vi "Detect PSw.vi"(4 "Contralateral Event Data":T1={"Event Data"={"LR"={"Phase"="LR", "On"=FALSE, "Last On Time"=0.0, "Duration"=0.0, "Crossing Time"=0.0, "Time since LR"=0.0, "Time Since TSw"=0.0, "Min gyro Z"=0.0, "Time since LR?"=FALSE, "Time since TSw?"=FALSE, "Min gyro Z?"=FALSE, "Crossing?"=FALSE}, "MSt"={"Phase"="MSt", "On"=FALSE, "Last On Time"=0.0, "Duration"=0.0}, "TSt"={"Phase"="TSt", "On"=FALSE, "Last On Time"=0.0, "Duration"=0.0}, "PSw"={"Phase"="PSw", "On"=FALSE, "Last On Time"=0.0, "Duration"=0.0}, "ISw"={"Phase"="ISw", "On"=FALSE, "Last On Time"=0.0, "Duration"=0.0, "Peak Time"=0.0, "Time since LR"=0.0, "Time since ISw"=0.0, "Time since LR?"=FALSE, "Time since ISw?"=FALSE, "Peak?"=FALSE}, "MSw"={"Phase"="MSw", "On"=FALSE, "Last On Time"=0.0, "Duration"=0.0, "Crossing time"=0.0, "Time since LR"=0.0, "Time since MSw"=0.0, "Time since ISw"=0.0, "Time since LR?"=FALSE, "Time since MSw?"=FALSE, "Time since ISw?"=FALSE, "Crossing?"=FALSE}, "TSw"={"Phase"="TSw", "On"=FALSE, "Last On Time"=0.0, "Duration"=0.0, "Peak time"=0.0, "Time since LR"=0.0, "Time since TSw"=0.0, "Time since LR?"=FALSE, "Time since TSw?"=FALSE, "Peak?"=FALSE}}, "Mean Cycle Duration"=0.0, "Event Detected?"=FALSE, "Last Event Detected"=0, "Num Cycles"=0.0, "GPD Log"=refnum, "Last Event Time"=0.0}, 5 "Ipsilateral Event Data":T1={"Event Data"={"LR"={"Phase"="LR", "On"=FALSE, "Last On Time"=0.0, "Duration"=0.0, "Crossing Time"=0.0, "Time since LR"=0.0, "Time Since TSw"=0.0, "Min gyro Z"=0.0, "Time since LR?"=FALSE, "Time since TSw?"=FALSE, "Min gyro Z?"=FALSE, "Crossing?"=FALSE}, "MSt"={"Phase"="MSt", "On"=FALSE, "Last On Time"=0.0, "Duration"=0.0}, "TSt"={"Phase"="TSt", "On"=FALSE, "Last On Time"=0.0, "Duration"=0.0}, "PSw"={"Phase"="PSw", "On"=FALSE, "Last On Time"=0.0, "Duration"=0.0}, "ISw"={"Phase"="ISw", "On"=FALSE, "Last On Time"=0.0, "Duration"=0.0, "Peak Time"=0.0, "Time since LR"=0.0, "Time since ISw"=0.0, "Time since LR?"=FALSE, "Time since ISw?"=FALSE, "Peak?"=FALSE}, "MSw"={"Phase"="MSw", "On"=FALSE, "Last On Time"=0.0, "Duration"=0.0, "Crossing time"=0.0, "Time since LR"=0.0, "Time since MSw"=0.0, "Time since ISw"=0.0, "Time since LR?"=FALSE, "Time since MSw?"=FALSE, "Time since ISw?"=FALSE, "Crossing?"=FALSE}, "TSw"={"Phase"="TSw", "On"=FALSE, "Last On Time"=0.0, "Duration"=0.0, "Peak time"=0.0, "Time since LR"=0.0, "Time since TSw"=0.0, "Time since LR?"=FALSE, "Time since TSw?"=FALSE, "Peak?"=FALSE}}, "Mean Cycle Duration"=0.0, "Event Detected?"=FALSE, "Last Event Detected"=0, "Num Cycles"=0.0, "GPD Log"=refnum, "Last Event Time"=0.0}) -> (1 "Contralateral Event Data":T1={"Event Data"={"LR"={"Phase"="LR", "On"=FALSE, "Last On Time"=0.0, "Duration"=0.0, "Crossing Time"=0.0, "Time since LR"=0.0, "Time Since TSw"=0.0, "Min gyro Z"=0.0, "Time since LR?"=FALSE, "Time since TSw?"=FALSE, "Min gyro Z?"=FALSE, "Crossing?"=FALSE}, "MSt"={"Phase"="MSt", "On"=FALSE, "Last On Time"=0.0, "Duration"=0.0}, "TSt"={"Phase"="TSt", "On"=FALSE, "Last On Time"=0.0, "Duration"=0.0}, "PSw"={"Phase"="PSw", "On"=FALSE, "Last On Time"=0.0, "Duration"=0.0}, "ISw"={"Phase"="ISw", "On"=FALSE, "Last On Time"=0.0, "Duration"=0.0, "Peak Time"=0.0, "Time since LR"=0.0, "Time since ISw"=0.0, "Time since LR?"=FALSE, "Time since ISw?"=FALSE, "Peak?"=FALSE}, "MSw"={"Phase"="MSw", "On"=FALSE, "Last On Time"=0.0, "Duration"=0.0, "Crossing time"=0.0, "Time since LR"=0.0, "Time since MSw"=0.0, "Time since ISw"=0.0, "Time since LR?"=FALSE, "Time since MSw?"=FALSE, "Time since ISw?"=FALSE, "Crossing?"=FALSE}, "TSw"={"Phase"="TSw", "On"=FALSE, "Last On Time"=0.0, "Duration"=0.0, "Peak time"=0.0, "Time since LR"=0.0, "Time since TSw"=0.0, "Time since LR?"=FALSE, "Time since TSw?"=FALSE, "Peak?"=FALSE}}, "Mean Cycle Duration"=0.0, "Event Detected?"=FALSE, "Last Event Detected"=0, "Num Cycles"=0.0, "GPD Log"=refnum, "Last Event Time"=0.0}, 2 "Ipsilateral Event Data":T1={"Event Data"={"LR"={"Phase"="LR", "On"=FALSE, "Last On Time"=0.0, "Duration"=0.0, "Crossing Time"=0.0, "Time since LR"=0.0, "Time Since TSw"=0.0, "Min gyro Z"=0.0, "Time since LR?"=FALSE, "Time since TSw?"=FALSE, "Min gyro Z?"=FALSE, "Crossing?"=FALSE}, "MSt"={"Phase"="MSt", "On"=FALSE, "Last On Time"=0.0, "Duration"=0.0}, "TSt"={"Phase"="TSt", "On"=FALSE, "Last On Time"=0.0, "Duration"=0.0}, "PSw"={"Phase"="PSw", "On"=FALSE, "Last On Time"=0.0, "Duration"=0.0}, "ISw"={"Phase"="ISw", "On"=FALSE, "Last On Time"=0.0, "Duration"=0.0, "Peak Time"=0.0, "Time since LR"=0.0, "Time since ISw"=0.0, "Time since LR?"=FALSE, "Time since ISw?"=FALSE, "Peak?"=FALSE}, "MSw"={"Phase"="MSw", "On"=FALSE, "Last On Time"=0.0, "Duration"=0.0, "Crossing time"=0.0, "Time since LR"=0.0, "Time since MSw"=0.0, "Time since ISw"=0.0, "Time since LR?"=FALSE, "Time since MSw?"=FALSE, "Time since ISw?"=FALSE, "Crossing?"=FALSE}, "TSw"={"Phase"="TSw", "On"=FALSE, "Last On Time"=0.0, "Duration"=0.0, "Peak time"=0.0, "Time since LR"=0.0, "Time since TSw"=0.0, "Time since LR?"=FALSE, "Time since TSw?"=FALSE, "Peak?"=FALSE}}, "Mean Cycle Duration"=0.0, "Event Detected?"=FALSE, "Last Event Detected"=0, "Num Cycles"=0.0, "GPD Log"=refnum, "Last Event Time"=0.0})   [LabVIEW 2019]
uses:
  Controls/Side Event Data.ctl
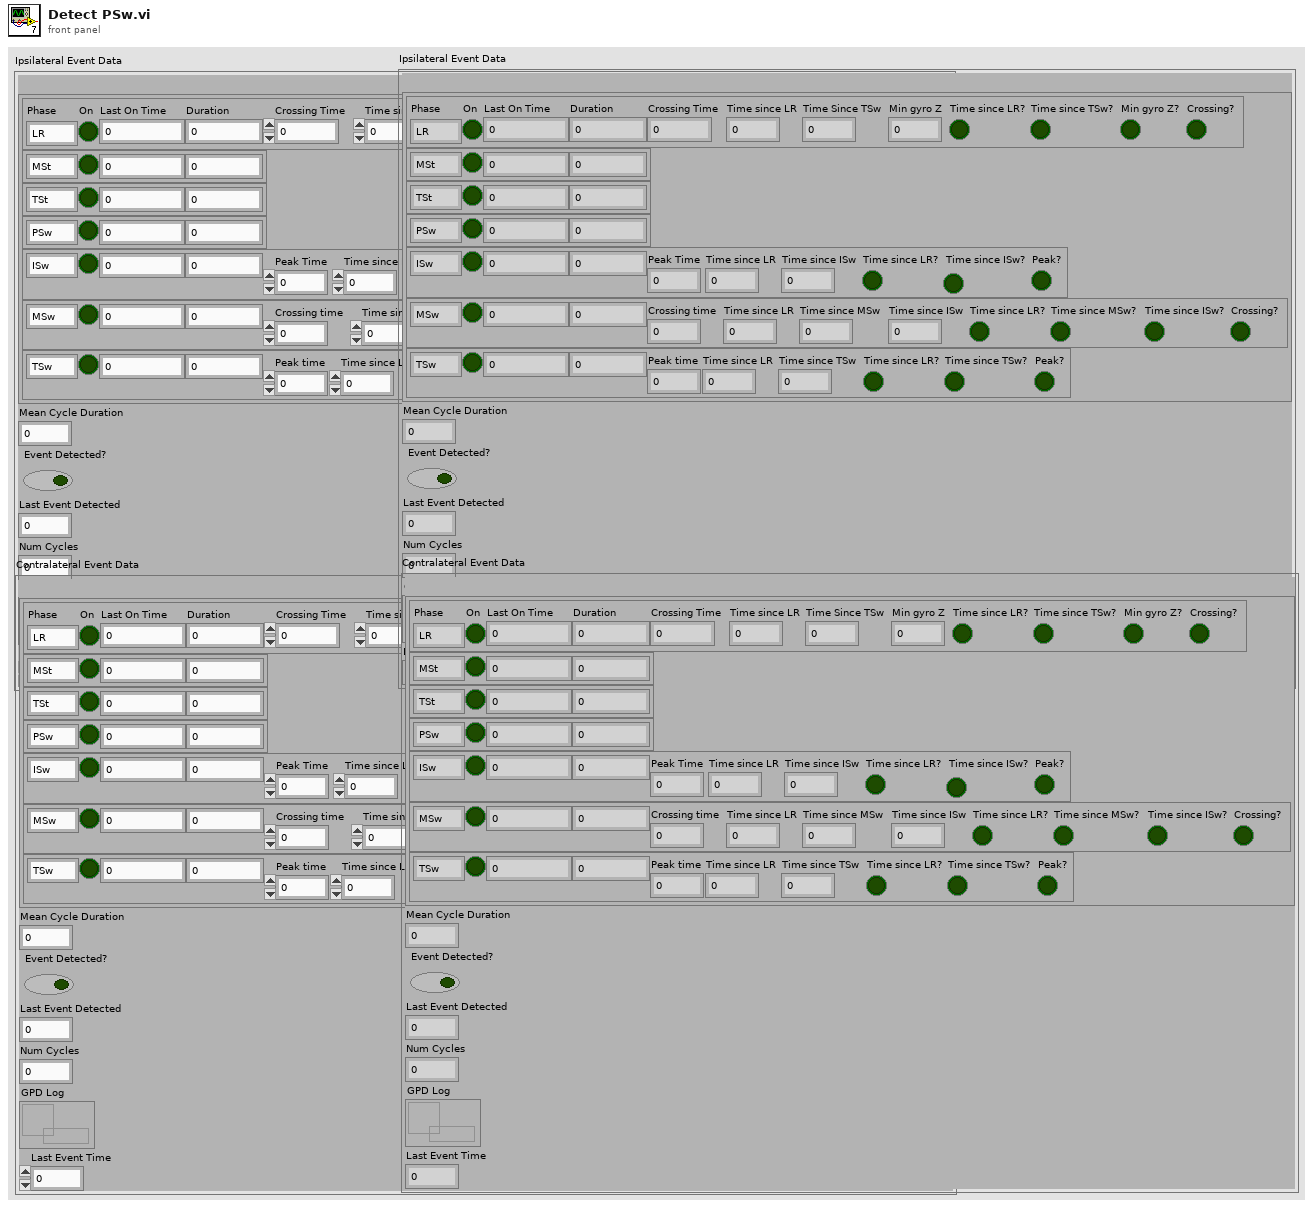
[diagram p1: front panel]
types:
  T1 = typedef "Side Event Data.ctl" = cluster{"Event Data":cluster{"LR":cluster{"Phase":string, "On":bool, "Last On Time":dbl, "Duration":dbl, "Crossing Time":dbl, "Time since LR":dbl, "Time Since TSw":dbl, "Min gyro Z":dbl, "Time since LR?":bool, "Time since TSw?":bool, "Min gyro Z?":bool, "Crossing?":bool}, "MSt":cluster{"Phase":string, "On":bool, "Last On Time":dbl, "Duration":dbl}, "TSt":cluster{"Phase":string, "On":bool, "Last On Time":dbl, "Duration":dbl}, "PSw":cluster{"Phase":string, "On":bool, "Last On Time":dbl, "Duration":dbl}, "ISw":cluster{"Phase":string, "On":bool, "Last On Time":dbl, "Duration":dbl, "Peak Time":dbl, "Time since LR":dbl, "Time since ISw":dbl, "Time since LR?":bool, "Time since ISw?":bool, "Peak?":bool}, "MSw":cluster{"Phase":string, "On":bool, "Last On Time":dbl, "Duration":dbl, "Crossing time":dbl, "Time since LR":dbl, "Time since MSw":dbl, "Time since ISw":dbl, "Time since LR?":bool, "Time since MSw?":bool, "Time since ISw?":bool, "Crossing?":bool}, "TSw":cluster{"Phase":string, "On":bool, "Last On Time":dbl, "Duration":dbl, "Peak time":dbl, "Time since LR":dbl, "Time since TSw":dbl, "Time since LR?":bool, "Time since TSw?":bool, "Peak?":bool}}, "Mean Cycle Duration":dbl, "Event Detected?":bool, "Last Event Detected":i32, "Num Cycles":dbl, "GPD Log":refnum<queue>, "Last Event Time":dbl}
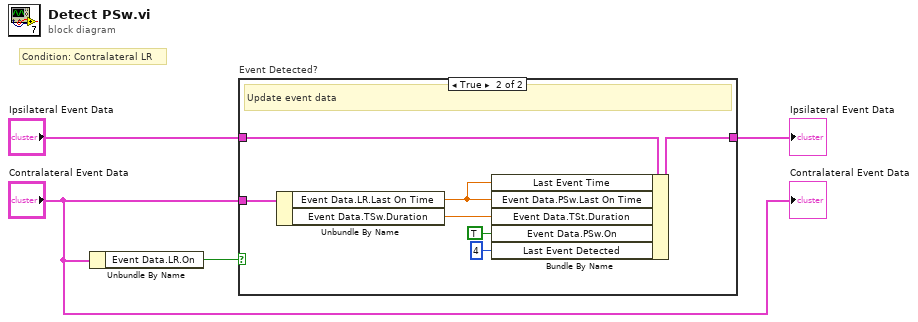
[diagram p0: block diagram]
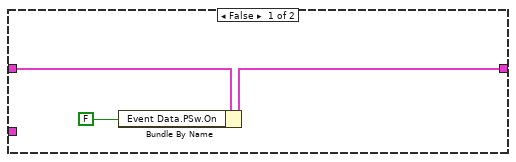
[diagram p2: hidden frame]
diagram:
  # "Condition: Contralateral LR"
  n1 = Unbundle By Name("Contralateral Event Data") -> ("Event Data.LR.On"=w4:bool)
  n2 = case "Event Detected?" shown="True" w4 {
    tunnel: [w5 w14] -> w1
    tunnel: "Ipsilateral Event Data" -> [w6 w12]
    tunnel: "Contralateral Event Data" -> [_ w13]
    frame False {
      n3 = Bundle By Name(cluster=w6, "Event Data.PSw.On"=FALSE) -> (w5:T1)
    }
    frame True {
      # "Update event data"
      n4 = Unbundle By Name(w13) -> ("Event Data.LR.Last On Time"=w8:dbl, "Event Data.TSw.Duration"=w11:dbl)
      n5 = Bundle By Name(cluster=w12, "Last Event Time"=w8, "Event Data.PSw.Last On Time"=w8, "Event Data.TSt.Duration"=w11, "Event Data.PSw.On"=TRUE, "Last Event Detected"=4) -> (w14:T1)
    }
  }
  "Ipsilateral Event Data" <- w1
  "Contralateral Event Data" <- "Contralateral Event Data"
